vi "keypress.vi"(8 "error in (no error)":errorcluster, 9 "VKey":T1, 10 "Char":i16, 11 "Worder in":refnum<class "Worder.lvclass">) -> (0 "error out":errorcluster, 3 "Worder out":refnum<class "Worder.lvclass">)   [LabVIEW 2020, in "Worder.lvclass"]
uses:
  Worder.lvclass
  letter_box.ctl
  <vilib>/event_ctls.llb/eventvkey.ctl
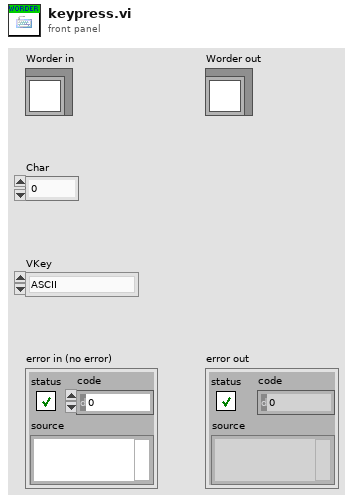
[diagram p1: front panel]
types:
  T1 = typedef "eventvkey.ctl" = enum16{"ASCII", "Enter", "Return", "Shift", "Ctrl", "Alt", "Cmd", "Opt", "Caps", "NumLock", "Clear", "Break", "Up", "Down", "Left", "Right", "Insert", "Delete", "Home", "End", "PageUp", "PageDown", "Escape", "Help", "Pause", "ScrollLock", "F1", "F2", "F3", "F4", "F5", "F6", "F7", "F8", "F9", "F10", "F11", "F12", "F13", "F14", "F15", "F16", "F17", "F18", "F19", "F20", "F21", "F22", "F23", "F24", "Play", "VolumeUp", "VolumeDown", "Mute", "Two Byte Char"}
  T2 = typedef "Worder.lvclass/letter_box.ctl" = cluster{"color":u32, "char":string}
  T3 = typedef "Worder.lvclass/keyboard.ctl" = cluster{"A":T4, "B":T4, "C":T4, "D":T4, "E":T4, "F":T4, "G":T4, "H":T4, "I":T4, "J":T4, "K":T4, "L":T4, "M":T4, "N":T4, "O":T4, "P":T4, "Q":T4, "R":T4, "S":T4, "T":T4, "U":T4, "V":T4, "W":T4, "X":T4, "Y":T4, "Z":T4}
  T4 = typedef "Worder.lvclass/letter_box_small.ctl" = cluster{"color":u32, "char":string}
  T5 = typedef "Worder.lvclass/config.ctl" = cluster{"num letters":i32, "num guesses":i32, "default color":u32, "match color":u32, "half match color":u32, "no match color":u32, "dictonary":string[]}
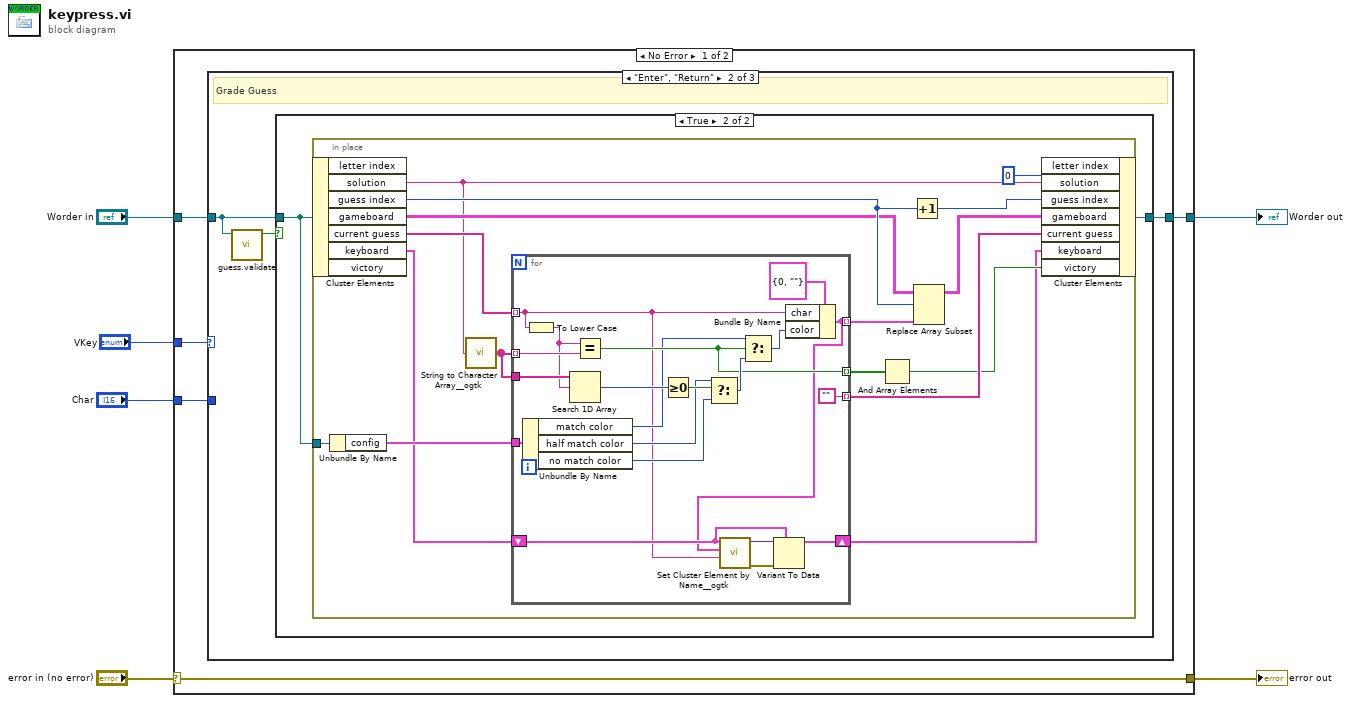
[diagram p0: block diagram]
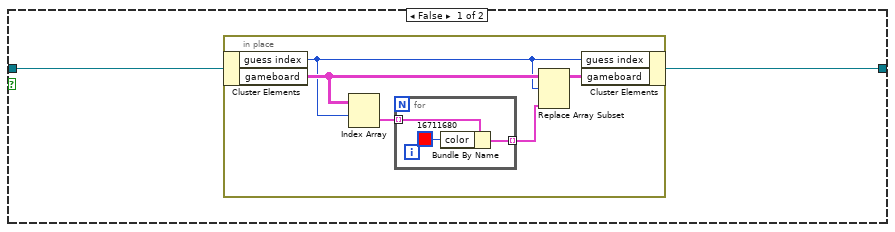
[diagram p3: hidden frame]
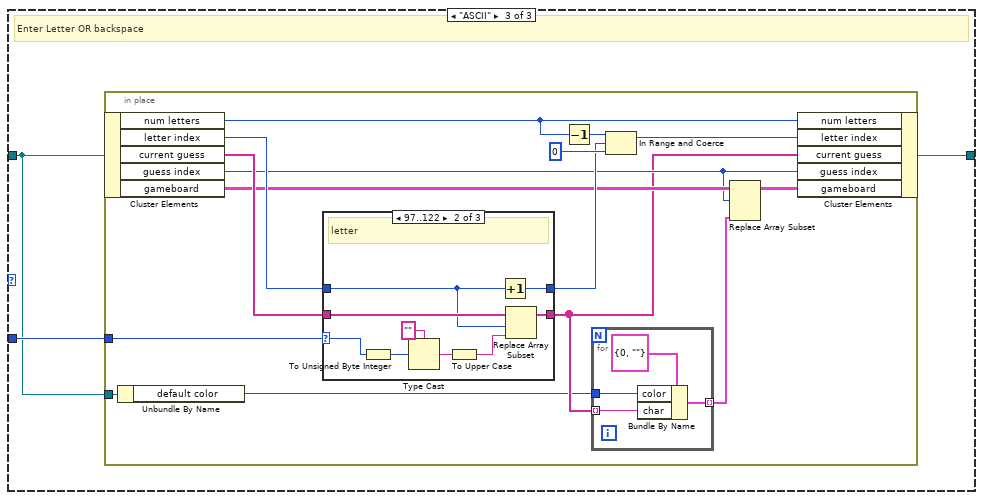
[diagram p4: hidden frame]
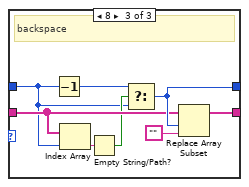
[diagram p6: hidden frame]
diagram:
  n1 = case shown="No Error" "error in (no error)" {
    selector: "error in (no error)" -> [w11 w106]
    tunnel: [w11 w106] -> w5
    tunnel: [w9 w105] -> w3
    tunnel: "Worder in" -> [w8 w105]
    tunnel: "Char" -> [w10 _]
    tunnel: "VKey" -> [w7 _]
    frame No Error {
      n2 = case shown="\"Enter\", \"Return\"" w7 {
        tunnel: w10 -> [_ _ w66]
        tunnel: [w12 w13 w65] -> w9
        tunnel: w8 -> [w12 w15 w64]
        frame Default {
        }
        frame "Enter", "Return" {
          # "Grade Guess"
          n3 = call "guess.validate.vi"("Worder in"=w15) -> ("valid?"=w14:bool)  [unwired: 10 in]
          n4 = case shown="True" w14 {
            tunnel: w15 -> [w17 w26]
            tunnel: [w16 w27] -> w13
            frame False {
              n5 = in-place {
                n6 = in-place-cluster #1(w17) -> ("guess index"=w19:i32, "gameboard"=w20:T2[][])
                n7 = Index Array(array=w20, index (row)=w19) -> (element=w18:T2[])  [unwired: 1 in]
                n8 = for {
                  tunnel: [w25] -> w22 mode=indexing
                  tunnel: w18 -> [w23] mode=indexing
                  n9 = Bundle By Name(cluster=w23, "color"=u32 16711680) -> (w25:T2)
                }
                n10 = Replace Array Subset(array=w20, new element=w22, index (row)=w19) -> (w21:T2[][])  [unwired: 1 in]
                n11 = in-place-cluster #1("guess index"=w19, "gameboard"=w21) -> (w16:refnum<class "Worder.lvclass">)
              }
            }
            frame True {
              n12 = in-place {
                in-place-border: w26 -> [w31]
                n13 = in-place-cluster #2(w26) -> ("solution"=w32:string, "guess index"=w41:i32, "gameboard"=w34:T2[][], "current guess"=w40:string[], "keyboard"=w29:T3)  [unwired: 2 out]
                n14 = Unbundle By Name(w31) -> ("config"=w30:T5)
                n15 = call "String to Character Array__ogtk.vi"("Input String"=w32) -> ("Character Array"=w42:string[])
                n16 = for {
                  tunnel: w42 -> [w63] mode=indexing
                  tunnel: w42 -> [w62]
                  tunnel: w40 -> [w44] mode=indexing
                  tunnel: [""] -> w38 mode=indexing
                  tunnel: [w45] -> w39 mode=indexing
                  tunnel: [w54] -> w37 mode=indexing
                  tunnel: w30 -> [w53]
                  shift-right: [w47] -> w28
                  shift-left: w29 -> [w48]
                  n17 = Unbundle By Name(w53) -> ("match color"=w52:u32, "half match color"=w50:u32, "no match color"=w51:u32)
                  n18 = To Lower Case(string=w44) -> (all lower case string=w58:string)
                  n19 = Search 1D Array(1D array=w62, element=w58) -> (index of element=w61:i32)  [unwired: 1 in]
                  n20 = Equal?(x=w58, y=w63) -> (x = y?=w54:bool)
                  n21 = Greater Or Equal To 0?(x=w61) -> (x >= 0?=w60:bool)
                  n22 = Select(t=w50, s=w60, f=w51) -> (s? t:f=w59:u32)
                  n23 = Select(t=w52, s=w54, f=w59) -> (s? t:f=w56:u32)
                  n24 = Bundle By Name(cluster=T2 {"color"=0, "char"=""} ("0"), "char"=w44, "color"=w56) -> (w45:T2)
                  n25 = call "Set Cluster Element by Name__ogtk.vi"("Element Name (\"\": New Element Data Name)"=w44, "New Element Value"=w45, "Cluster"=w48) -> ("error out"=w46:errorcluster, "VCluster out"=w49:variant)  [unwired: 6 in, 1 out]
                  n26 = Variant To Data(error in=w46, type=w48, Variant=w49) -> (data=w47:T3)  [unwired: 1 out]
                }
                n27 = And Array Elements(Boolean array=w37) -> (logical AND=w36:bool)
                n28 = Increment(x=w41) -> (x+1=w43:i32)
                n29 = Replace Array Subset(array=w34, new element=w39, index (row)=w41) -> (w33:T2[][])  [unwired: 1 in]
                n30 = in-place-cluster #2("letter index"=0, "solution"=w32, "guess index"=w43, "gameboard"=w33, "current guess"=w38, "keyboard"=w28, "victory"=w36) -> (w27:refnum<class "Worder.lvclass">)
              }
            }
          }
        }
        frame "ASCII" {
          # "Enter Letter OR backspace"
          n31 = in-place {
            in-place-border: w66 -> [w76]
            in-place-border: w64 -> [w68]
            n32 = in-place-cluster #3(w64) -> ("num letters"=w69:i32, "letter index"=w81:i32, "current guess"=w77:string[], "guess index"=w73:i32, "gameboard"=w74:T2[][])
            n33 = Unbundle By Name(w68) -> ("default color"=w67:u32)
            n34 = case shown="97..122" w76 {
              selector: w76 -> [_ w93 _]
              tunnel: w81 -> [w87 w88 w97]
              tunnel: [w87 w96 w101] -> w79
              tunnel: w77 -> [w86 w91 w100]
              tunnel: [w86 w90 w104] -> w72
              frame Default {
              }
              frame 97..122 {
                # "letter"
                n35 = To Unsigned Byte Integer(number=w93) -> (unsigned 8bit integer=w92:u8)
                n36 = Type Cast(type="", x=w92) -> (*(type *) &x=w95:string)
                n37 = To Upper Case(1:w95) -> (0:w89:string)
                n38 = Increment(x=w88) -> (x+1=w96:i32)
                n39 = Replace Array Subset(array=w91, new element=w89, index=w88) -> (w90:string[])
              }
              frame 8 {
                # "backspace"
                n40 = Decrement(x=w97) -> (x-1=w102:i32)
                n41 = Index Array(array=w100, index=w97) -> (element=w99:string)
                n42 = Empty String/Path?(string/path=w99) -> (empty?=w98:bool)
                n43 = Select(t=w102, s=w98, f=w97) -> (s? t:f=w101:i32)
                n44 = Replace Array Subset(array=w100, new element="", index=w101) -> (w104:string[])
              }
            }
            n45 = Decrement(x=w69) -> (x-1=w75:i32)
            n46 = for {
              tunnel: w67 -> [w83]
              tunnel: w72 -> [w82] mode=indexing
              tunnel: [w84] -> w71 mode=indexing
              n47 = Bundle By Name(cluster=T2 {"color"=0, "char"=""} ("0"), "color"=w83, "char"=w82) -> (w84:T2)
            }
            n48 = In Range and Coerce(upper limit=w75, x=w79, lower limit=0) -> (coerced(x)=w78:i32)  [unwired: 1 out]
            n49 = Replace Array Subset(array=w74, new element=w71, index (row)=w73) -> (w70:T2[][])  [unwired: 1 in]
            n50 = in-place-cluster #3("num letters"=w69, "letter index"=w78, "current guess"=w72, "guess index"=w73, "gameboard"=w70) -> (w65:refnum<class "Worder.lvclass">)
          }
        }
      }
    }
    frame Error {
    }
  }
  "error out" <- w5
  "Worder out" <- w3
